vi "Process.vi"(11 "Actor":refnum<class "Process Input View.lvclass">) -> ()   [LabVIEW 2015, in "Process Input View.lvclass"]
uses:
  Process Input View.lvclass
  Re-use Libraries/Minimal Actor Framework/Actors/Base Actor/Actor/Front Panel State.ctl
  Re-use Libraries/Minimal Actor Framework/Actors/Base Actor/Actor/Actor.lvclass
  Re-use Libraries/Minimal Actor Framework/Messaging/Message/Message.lvclass
  Actors/Alarm Handler/API/Alarm Handler Actor API.lvclass
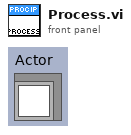
[diagram p1: front panel]
types:
  T1 = typedef "Actor.lvclass/Front Panel State.ctl" = enum32{"Invalid", "Standard", "Closed", "Hidden", "Minimized", "Maximized"}
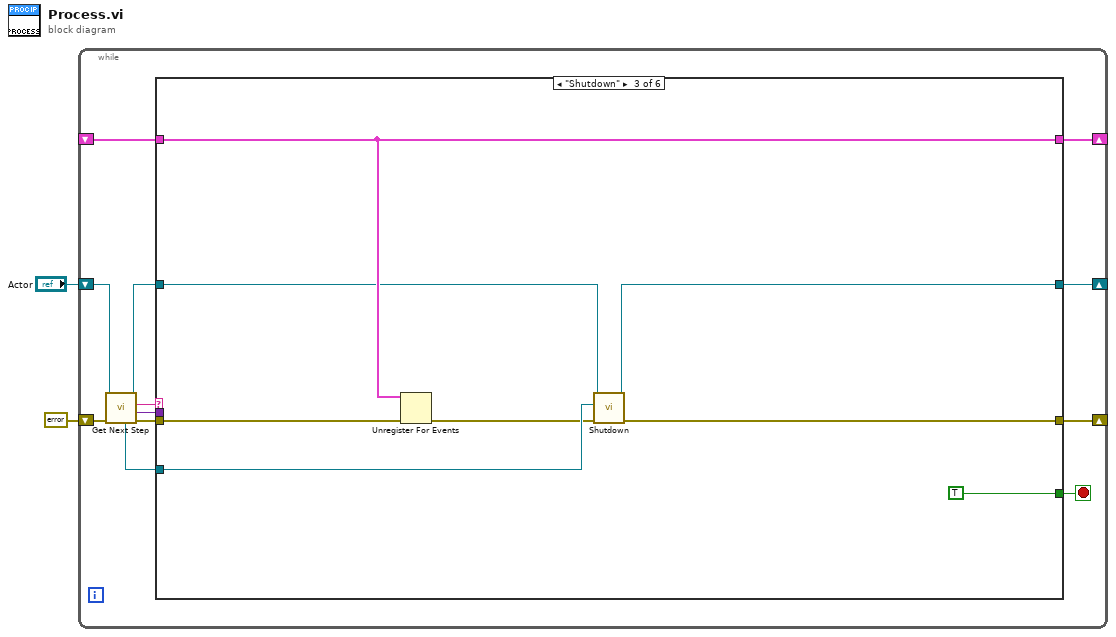
[diagram p0: block diagram]
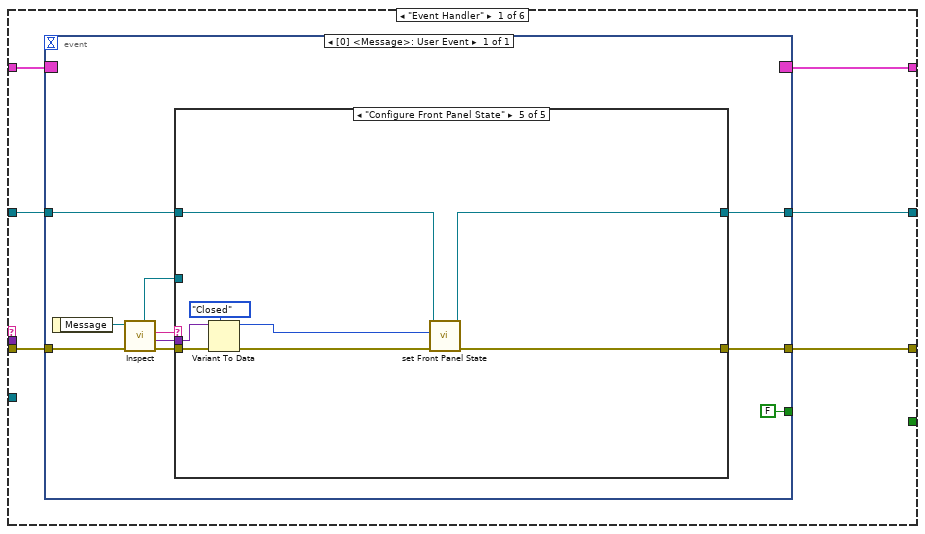
[diagram p2: hidden frame]
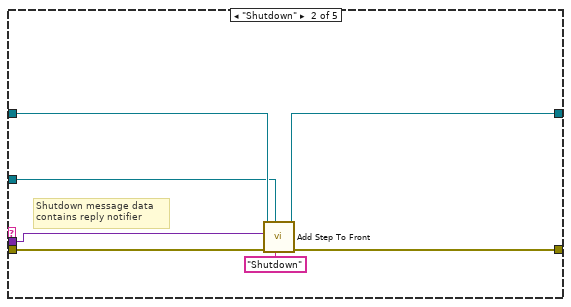
[diagram p4: hidden frame]
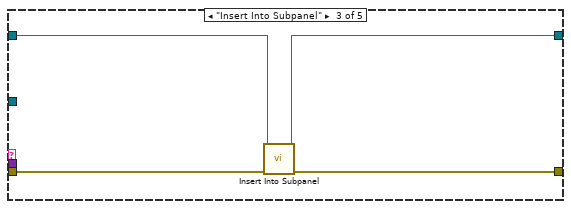
[diagram p5: hidden frame]
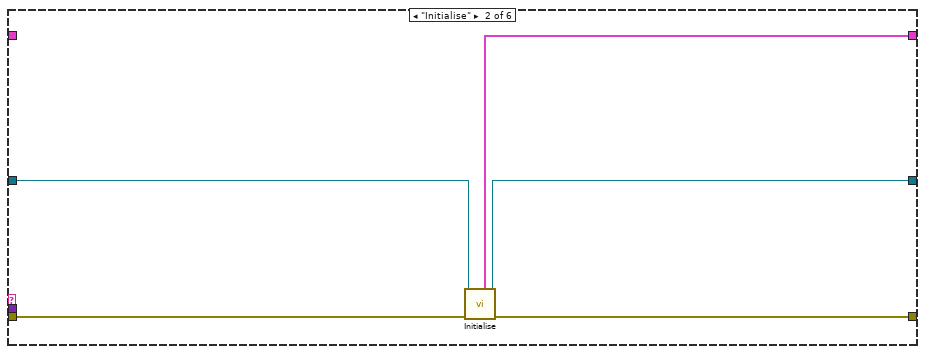
[diagram p7: hidden frame]
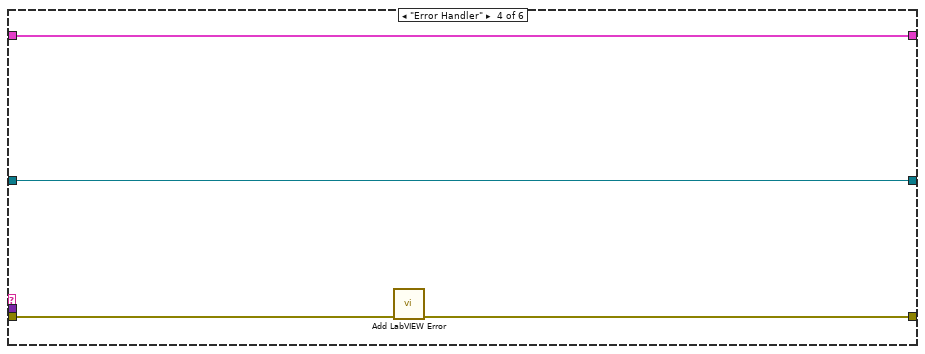
[diagram p8: hidden frame]
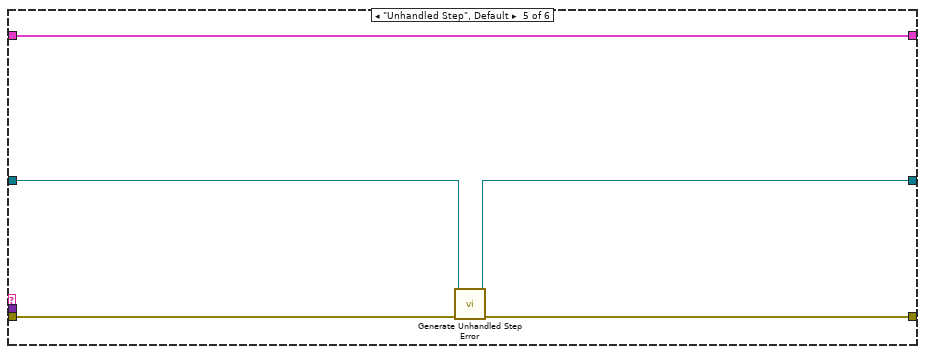
[diagram p9: hidden frame]
diagram:
  n1 = while {
    shift-right: [w5] -> _
    shift-left: "Actor" -> [w13]
    shift-right: [w10] -> _
    shift-left: _ -> [w9]
    shift-right: [w4] -> _
    shift-left: errorcluster {"status"=FALSE, "code"=0, "source"=""} ("error constant") -> [w7]
    stop <- w14 stop-if-true
    n2 = call-dynamic "Get Next Step.vi"("error in (no error)"=w7, "Actor in"=w13) -> ("error out"=w8:errorcluster, "Parameter"=w11:variant, "Step"=w6:string, "Actor out"=w12:refnum<class "Process Input View.lvclass">, "Reply Channel"=w3:refnum<notifier>)  [unwired: 5 in]
    n3 = case shown="\"Shutdown\"" w6 {
      tunnel: [_ _ TRUE _ _ _] -> w14
      tunnel: w12 -> [w20 w55 w63 w67 w74 w77]
      tunnel: [w19 w56 w62 w67 w73 w77] -> w5
      tunnel: w11 -> [_ _ _ _ _ _]
      tunnel: [w17 w58 w65 w70 w75 w78] -> w10
      tunnel: w9 -> [w18 _ w65 w70 w75 w78]
      tunnel: w8 -> [w16 w54 w64 w69 w72 w76]
      tunnel: [w15 w57 w59 w68 w71 w76] -> w4
      tunnel: w3 -> [_ _ w61 _ _ _]
      frame "Event Handler" {
        n4 = event shown="[0] <Message>: User Event" {
          selector: w18 -> [_]
          dyn-events: [_] -> w17
          timeout: _ -> [_]
          tunnel: w20 -> [w30]
          tunnel: [w29] -> w19
          tunnel: w16 -> [w27]
          tunnel: [w28] -> w15
          tunnel: [FALSE] -> _
          event User Event {
            n5 = event-data() -> ("Message"=w26:refnum<class "Message.lvclass">)  [unwired: 1 in]
            n6 = call "Inspect.vi"("error in (no error)"=w27, "Message in"=w26) -> ("error out"=w23:errorcluster, "Data"=w24:variant, "Name"=w25:string, "Reply Channel"=w22:refnum<notifier>)  [unwired: 5 in, 1 out]
            n7 = case shown="\"Configure Front Panel State\"" w25 {
              tunnel: w30 -> [w32 w39 w43 w44 w53]
              tunnel: [w32 w38 w42 w44 w52] -> w29
              tunnel: w23 -> [w31 w36 w41 w45 w49]
              tunnel: [w31 w35 w40 w45 w51] -> w28
              tunnel: w24 -> [_ w34 _ _ w50]
              tunnel: w22 -> [_ w33 _ _ _]
              frame Default {
              }
              frame "Shutdown" {
                # "Shutdown message data contains reply notifier"
                n8 = call-dynamic "Add Step To Front.vi"("Step Name"="Shutdown", "Reply Channel"=w33, "error in (no error)"=w36, "Parameter"=w34, "Actor in"=w39) -> ("error out"=w35:errorcluster, "Actor out"=w38:refnum<class "Process Input View.lvclass">)  [unwired: 5 in]
              }
              frame "Insert Into Subpanel" {
                n9 = call-dynamic "Insert Into Subpanel.vi"("error in (no error)"=w41, "Actor in"=w43) -> ("error out"=w40:errorcluster, "Actor out"=w42:refnum<class "Process Input View.lvclass">)  [unwired: 8 in]
              }
              frame "State Update Tick" {
                # "Called by the Metronome"
              }
              frame "Configure Front Panel State" {
                n10 = Variant To Data(error in=w49, type=Front_Panel_State."Closed" ("Front Panel State"), Variant=w50) -> (data=w46:T1, error out=w48:errorcluster)
                n11 = call-dynamic "set Front Panel State.vi"("error in (no error)"=w48, "Front Panel State"=w46, "Actor in"=w53) -> ("error out"=w51:errorcluster, "Actor out"=w52:refnum<class "Process Input View.lvclass">)  [unwired: 7 in]
              }
            }
          }
        }
      }
      frame "Initialise" {
        n12 = call "Initialise.vi"("error in (no error)"=w54, "Actor in"=w55) -> ("error out"=w57:errorcluster, "Actor out"=w56:refnum<class "Process Input View.lvclass">, "Observers"=w58:cluster{"Actor":refnum<event-registration>})  [unwired: 7 in]
      }
      frame "Shutdown" {
        n13 = Unregister For Events(event registration refnum=w65, error in=w64) -> (error out=w60:errorcluster)
        n14 = call-dynamic "Shutdown.vi"("error in (no error)"=w60, "Reply Channel"=w61, "Actor in"=w63) -> ("error out"=w59:errorcluster, "Actor out"=w62:refnum<class "Process Input View.lvclass">)  [unwired: 7 in]
      }
      frame "Error Handler" {
        n15 = call "Add LabVIEW Error.vi"("error in (no error)"=w69) -> ("error out"=w68:errorcluster)  [unwired: 10 in]
      }
      frame "Unhandled Step", Default {
        n16 = call-dynamic "Generate Unhandled Step Error.vi"("error in (no error)"=w72, "Actor in"=w74) -> ("error out"=w71:errorcluster, "Actor out"=w73:refnum<class "Process Input View.lvclass">)  [unwired: 8 in]
      }
      frame "-----------------------" {
        # "Separator"
      }
    }
  }
